vi "Reference to Parent.vi"(8 "error in (no error)":errorcluster) -> (0 "error out":errorcluster, 3 "Parent Reference":refnum<vi>)   [LabVIEW 2011]
doc: "Gets reference to the parent VI.\n\n\nVersion 1.0 - 2/14/2013\n\nPhaeron, Inc.\nwww.phaeron.com\ninfo@phaeron.com"
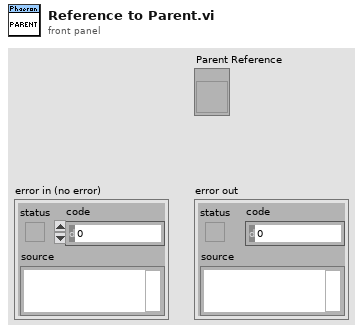
[diagram p1: front panel]
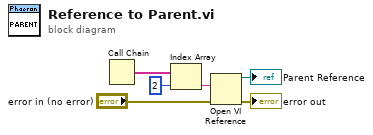
[diagram p0: block diagram]
diagram:
  n1 = Call Chain() -> (call chain=w6:string[])
  n2 = Index Array(array=w6, index=2) -> (element=w4:string)
  n3 = Open VI Reference(vi path=w4, error in (no error)="error in (no error)") -> (vi reference=→"Parent Reference":refnum<vi>, error out=→"error out":errorcluster)  [unwired: 4 in]
